vi "Make File Tree.vi"(8 "Error In":errorcluster, 10 "TreeControl in":refnum<vi>, 11 "WAD Main Cluster":T1) -> (0 "Error Out":errorcluster, 2 "TreeControl OUT":refnum<vi>, 3 "WAD Main Cluster OUT":T1)   [LabVIEW 2017]
uses:
  WAD_MainCluster.ctl
  TextureList.ctl
  PatchList.ctl
  Lumps.ctl
  <userlib>/_OpenG.lib/array/array.llb/Remove Duplicates from 1D Array (String)__ogtk.vi
  <userlib>/_OpenG.lib/array/array.llb/Filter 1D Array (String)__ogtk.vi
  <vilib>/regexp/Match Regular Expression.xnode
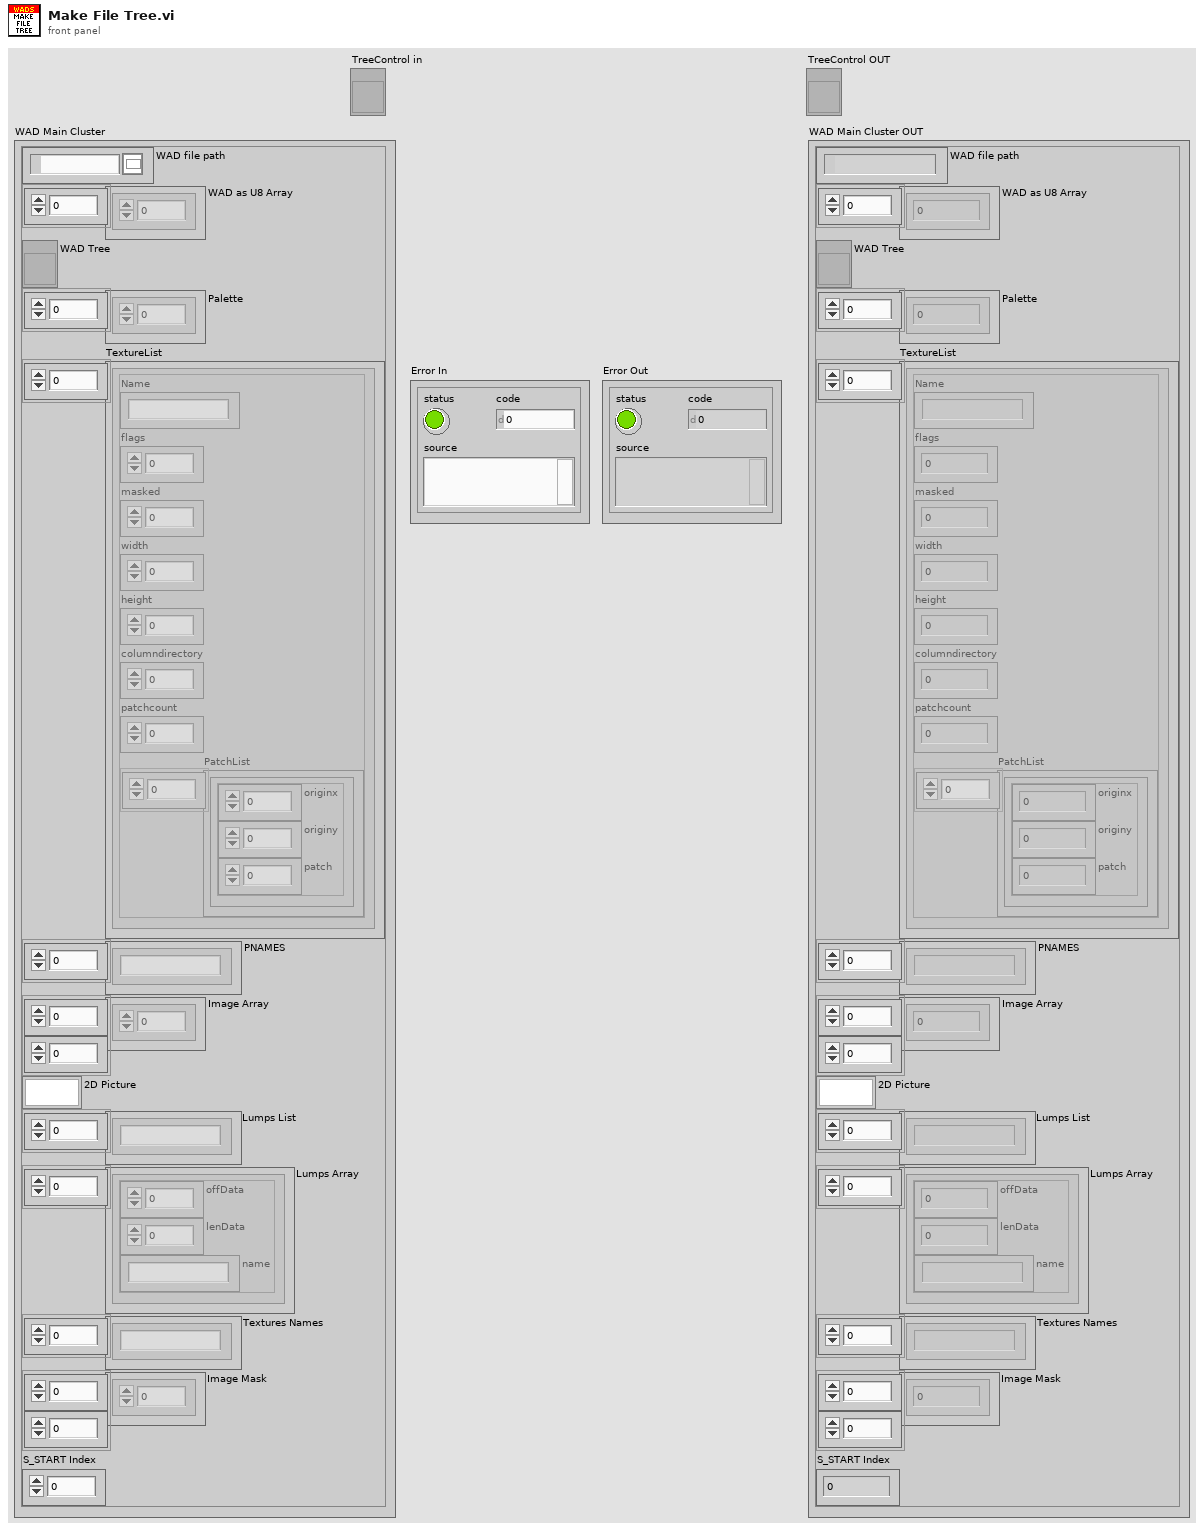
[diagram p1: front panel]
types:
  T1 = typedef "WAD_MainCluster.ctl" = cluster{"WAD file path":path, "WAD as U8 Array":u8[], "WAD Tree":refnum<vi>, "Palette":u32[], "TextureList":T2[], "PNAMES":string[], "Image Array":i16[][], "2D Picture":picture, "Lumps List":string[], "Lumps Array":T4[], "Textures Names":string[], "Image Mask":i16[][], "S_START Index":i32}
  T2 = typedef "TextureList.ctl" = cluster{"Name":string, "flags":u16, "masked":i16, "width":i16, "height":i16, "columndirectory":u32, "patchcount":i16, "PatchList":T3[]}
  T3 = typedef "PatchList.ctl" = cluster{"originx":i16, "originy":i16, "patch":i16}
  T4 = typedef "Lumps.ctl" = cluster{"offData":i32, "lenData":i32, "name":string}
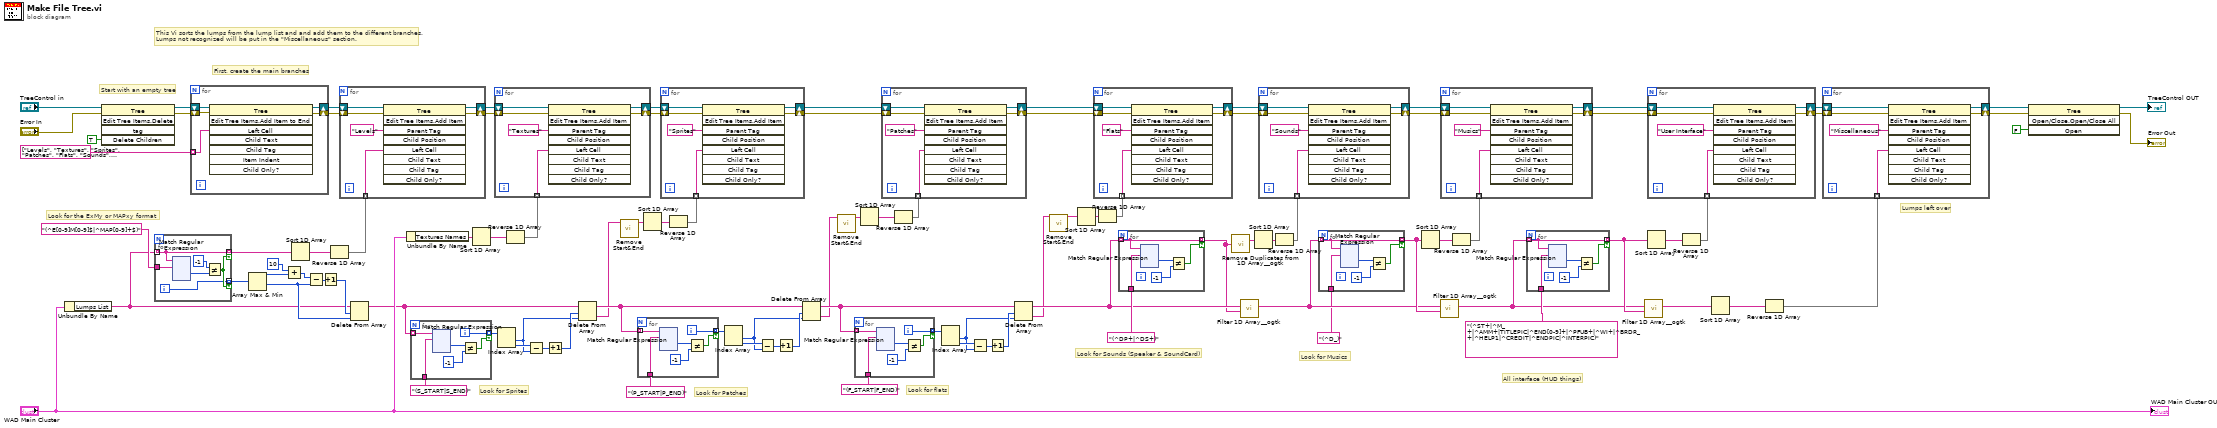
[diagram p0: block diagram]
diagram:
  # "This Vi sorts the lumps from the lump list and and add them to the different branches.\nLumps not recognized will be put in the \"Miscellaneous\" section."
  # "Start with an empty tree"
  # "First, create the main branches"
  # "Look for Musics"
  # "Lumps left over"
  # "All interface (HUD things)"
  # "Look for Sounds (Speaker & SoundCard)"
  # "Look for Sprites"
  # "Look for Patches"
  # "Look for flats"
  # "Look for the ExMy or MAPxy format"
  n1 = Unbundle By Name("WAD Main Cluster") -> ("Lumps List"=w5:string[])
  n2 = invoke on="Invoke Node" class="Tree" method="Edit Tree Items.Delete"(reference="TreeControl in", error in="Error In", "Delete Children"=TRUE ("Delete Children?")) -> (reference out=w90:refnum<vi>, error out=w92:errorcluster)  [unwired: 2 in, 3 out]
  n3 = for {
    tunnel: w5 -> [w101] mode=indexing
    tunnel: "(^E[0-9]M[0-9]$|^MAP[0-9]+$)" ("format string") -> [w102]
    tunnel: [w101] -> w83 mode=indexing if=w99
    tunnel: [w98] -> w65 mode=indexing if=w99
    i -> [w98]
    n4 = xnode "Match Regular Expression"("input string"=w101, "regular expression"=w102) -> ("offset past match"=w100:i32)  [unwired: 4 in, 4 out]
    n5 = Not Equal?(x=-1, y=w100) -> (x != y?=w99:bool)
  }
  n6 = for {
    tunnel: string[] ["Levels", "Textures", "Sprites", "Patches", "Flats", "Sounds", "Musics", "User Interface", "Miscellaneous"] -> [w220] mode=indexing
    shift-right: [w221] -> w93
    shift-left: w92 -> [w222]
    shift-right: [w218] -> w89
    shift-left: w90 -> [w219]
    n7 = invoke on="Invoke Node" class="Tree" method="Edit Tree Items.Add Item to End"(reference=w219, error in=w222, "Left Cell"=w220) -> (reference out=w218:refnum<vi>, error out=w221:errorcluster)  [unwired: 5 in, 6 out]
  }
  n8 = Array Max & Min(array=w65) -> (max value=w64:i32, min value=w61:i32)  [unwired: 2 out]
  n9 = Add(x=10, y=w64) -> (x+y=w62:i32)
  n10 = Sort 1D Array(array=w83) -> (sorted array=w14:string[])
  n11 = Subtract(x=w62, y=w61) -> (x-y=w60:i32)
  n12 = Increment(x=w60) -> (x+1=w59:i32)
  n13 = Reverse 1D Array(array=w14) -> (reversed array=w94:string[])
  n14 = for {
    tunnel: w94 -> [w223] mode=indexing
    shift-right: [w226] -> w32
    shift-left: w93 -> [w228]
    shift-right: [w224] -> w33
    shift-left: w89 -> [w225]
    n15 = invoke on="Invoke Node" class="Tree" method="Edit Tree Items.Add Item"(reference=w225, error in=w228, "Parent Tag"="Levels", "Left Cell"=w223) -> (reference out=w224:refnum<vi>, error out=w226:errorcluster)  [unwired: 5 in, 7 out]
  }
  n16 = Delete From Array(array=w5, length=w59, index=w61) -> (array with subset deleted=w58:string[])  [unwired: 1 out]
  n17 = Unbundle By Name("WAD Main Cluster") -> ("Textures Names"=w86:string[])
  n18 = for {
    tunnel: w58 -> [w231] mode=indexing
    tunnel: "(S_START|S_END)" ("format string") -> [w232]
    tunnel: [w229] -> w71 mode=indexing if=w230
    i -> [w229]
    n19 = xnode "Match Regular Expression"("input string"=w231, "regular expression"=w232) -> ("offset past match"=w234:i32)  [unwired: 4 in, 4 out]
    n20 = Not Equal?(x=w234, y=-1) -> (x != y?=w230:bool)
  }
  n21 = Sort 1D Array(array=w86) -> (sorted array=w13:string[])
  n22 = Index Array(array=w71) -> (element #1=w38:i32, element #2=w70:i32)  [unwired: 2 in]
  n23 = Reverse 1D Array(array=w13) -> (reversed array=w96:string[])
  n24 = for {
    shift-right: [w352] -> w30
    shift-left: w32 -> [w354]
    tunnel: w96 -> [w351] mode=indexing
    shift-right: [w349] -> w31
    shift-left: w33 -> [w350]
    n25 = invoke on="Invoke Node" class="Tree" method="Edit Tree Items.Add Item"(reference=w350, error in=w354, "Parent Tag"="Textures", "Left Cell"=w351) -> (reference out=w349:refnum<vi>, error out=w352:errorcluster)  [unwired: 5 in, 7 out]
  }
  n26 = Subtract(x=w70, y=w38) -> (x-y=w68:i32)
  n27 = Increment(x=w68) -> (x+1=w57:i32)
  n28 = Delete From Array(array=w58, length=w57, index=w38) -> (deleted portion=w27:string[], array with subset deleted=w56:string[])
  n29 = call "Remove Start&End.vi"("Lumps List"=w27) -> ("filtered array"=w26:string[])  [unwired: 10 in]
  n30 = for {
    tunnel: w56 -> [w357] mode=indexing
    tunnel: "(P_START|P_END)" ("format string") -> [w358]
    tunnel: [w355] -> w76 mode=indexing if=w356
    i -> [w355]
    n31 = xnode "Match Regular Expression"("input string"=w357, "regular expression"=w358) -> ("offset past match"=w360:i32)  [unwired: 4 in, 4 out]
    n32 = Not Equal?(x=w360, y=-1) -> (x != y?=w356:bool)
  }
  n33 = Sort 1D Array(array=w26) -> (sorted array=w12:string[])
  n34 = Reverse 1D Array(array=w12) -> (reversed array=w67:string[])
  n35 = for {
    shift-right: [w478] -> w24
    shift-left: w30 -> [w480]
    tunnel: w67 -> [w477] mode=indexing
    shift-right: [w475] -> w25
    shift-left: w31 -> [w476]
    n36 = invoke on="Invoke Node" class="Tree" method="Edit Tree Items.Add Item"(reference=w476, error in=w480, "Parent Tag"="Sprites", "Left Cell"=w477) -> (reference out=w475:refnum<vi>, error out=w478:errorcluster)  [unwired: 5 in, 7 out]
  }
  n37 = Index Array(array=w76) -> (element #1=w37:i32, element #2=w77:i32)  [unwired: 2 in]
  n38 = Subtract(x=w77, y=w37) -> (x-y=w74:i32)
  n39 = Increment(x=w74) -> (x+1=w46:i32)
  n40 = Delete From Array(array=w56, length=w46, index=w37) -> (deleted portion=w35:string[], array with subset deleted=w49:string[])
  n41 = call "Remove Start&End.vi"("Lumps List"=w35) -> ("filtered array"=w34:string[])  [unwired: 10 in]
  n42 = for {
    tunnel: w49 -> [w483] mode=indexing
    tunnel: "(F_START|F_END)" ("format string") -> [w484]
    tunnel: [w481] -> w81 mode=indexing if=w482
    i -> [w481]
    n43 = xnode "Match Regular Expression"("input string"=w483, "regular expression"=w484) -> ("offset past match"=w486:i32)  [unwired: 4 in, 4 out]
    n44 = Not Equal?(x=w486, y=-1) -> (x != y?=w482:bool)
  }
  n45 = Sort 1D Array(array=w34) -> (sorted array=w11:string[])
  n46 = Reverse 1D Array(array=w11) -> (reversed array=w73:string[])
  n47 = for {
    shift-right: [w604] -> w54
    shift-left: w24 -> [w606]
    tunnel: w73 -> [w603] mode=indexing
    shift-right: [w601] -> w55
    shift-left: w25 -> [w602]
    n48 = invoke on="Invoke Node" class="Tree" method="Edit Tree Items.Add Item"(reference=w602, error in=w606, "Parent Tag"="Patches", "Left Cell"=w603) -> (reference out=w601:refnum<vi>, error out=w604:errorcluster)  [unwired: 5 in, 7 out]
  }
  n49 = Index Array(array=w81) -> (element #1=w36:i32, element #2=w80:i32)  [unwired: 2 in]
  n50 = Subtract(x=w80, y=w36) -> (x-y=w79:i32)
  n51 = Increment(x=w79) -> (x+1=w47:i32)
  n52 = Delete From Array(array=w49, length=w47, index=w36) -> (deleted portion=w29:string[], array with subset deleted=w40:string[])
  n53 = call "Remove Start&End.vi"("Lumps List"=w29) -> ("filtered array"=w28:string[])  [unwired: 10 in]
  n54 = Sort 1D Array(array=w28) -> (sorted array=w10:string[])
  n55 = Reverse 1D Array(array=w10) -> (reversed array=w78:string[])
  n56 = for {
    shift-right: [w610] -> w52
    shift-left: w54 -> [w612]
    tunnel: w78 -> [w609] mode=indexing
    shift-right: [w607] -> w53
    shift-left: w55 -> [w608]
    n57 = invoke on="Invoke Node" class="Tree" method="Edit Tree Items.Add Item"(reference=w608, error in=w612, "Parent Tag"="Flats", "Left Cell"=w609) -> (reference out=w607:refnum<vi>, error out=w610:errorcluster)  [unwired: 5 in, 7 out]
  }
  n58 = for {
    tunnel: w40 -> [w614] mode=indexing
    tunnel: "(^DP+|^DS+)" ("format string") -> [w615]
    tunnel: [w614] -> w3 mode=indexing if=w613
    n59 = xnode "Match Regular Expression"("input string"=w614, "regular expression"=w615) -> ("offset past match"=w617:i32)  [unwired: 4 in, 4 out]
    n60 = Not Equal?(x=w617, y=-1) -> (x != y?=w613:bool)
  }
  n61 = call-poly <userlib>:"Remove Duplicates from 1D Array__ogtk.vi"("Input Array"=w3) -> ("Output Array"=w2:string[])  [unwired: 1 out]
  n62 = call-poly <userlib>:"Filter 1D Array__ogtk.vi"("items to filter"=w3, "array"=w40) -> ("filtered array"=w22:string[])  [unwired: 4 in, 1 out]
  n63 = Sort 1D Array(array=w2) -> (sorted array=w9:string[])
  n64 = Reverse 1D Array(array=w9) -> (reversed array=w4:string[])
  n65 = for {
    shift-right: [w735] -> w19
    shift-left: w52 -> [w737]
    tunnel: w4 -> [w734] mode=indexing
    shift-right: [w732] -> w20
    shift-left: w53 -> [w733]
    n66 = invoke on="Invoke Node" class="Tree" method="Edit Tree Items.Add Item"(reference=w733, error in=w737, "Parent Tag"="Sounds", "Left Cell"=w734) -> (reference out=w732:refnum<vi>, error out=w735:errorcluster)  [unwired: 5 in, 7 out]
  }
  n67 = for {
    tunnel: w22 -> [w739] mode=indexing
    tunnel: "(^D_)" ("format string") -> [w740]
    tunnel: [w739] -> w23 mode=indexing if=w738
    n68 = xnode "Match Regular Expression"("input string"=w739, "regular expression"=w740) -> ("offset past match"=w742:i32)  [unwired: 4 in, 4 out]
    n69 = Not Equal?(x=w742, y=-1) -> (x != y?=w738:bool)
  }
  n70 = Sort 1D Array(array=w23) -> (sorted array=w8:string[])
  n71 = call-poly <userlib>:"Filter 1D Array__ogtk.vi"("items to filter"=w23, "array"=w22) -> ("filtered array"=w15:string[])  [unwired: 4 in, 1 out]
  n72 = Reverse 1D Array(array=w8) -> (reversed array=w16:string[])
  n73 = for {
    shift-right: [w860] -> w17
    shift-left: w19 -> [w862]
    tunnel: w16 -> [w859] mode=indexing
    shift-right: [w857] -> w18
    shift-left: w20 -> [w858]
    n74 = invoke on="Invoke Node" class="Tree" method="Edit Tree Items.Add Item"(reference=w858, error in=w862, "Parent Tag"="Musics", "Left Cell"=w859) -> (reference out=w857:refnum<vi>, error out=w860:errorcluster)  [unwired: 5 in, 7 out]
  }
  n75 = for {
    tunnel: w15 -> [w864] mode=indexing
    tunnel: "(^ST+|^M_+|^AMM+|TITLEPIC|^END[0-9]+|^PFUB+|^WI+|^BRDR_+|^HELP1|^CREDIT|^ENDPIC|^INTERPIC)" ("format string") -> [w865]
    tunnel: [w864] -> w39 mode=indexing if=w863
    n76 = xnode "Match Regular Expression"("input string"=w864, "regular expression"=w865) -> ("offset past match"=w867:i32)  [unwired: 4 in, 4 out]
    n77 = Not Equal?(x=w867, y=-1) -> (x != y?=w863:bool)
  }
  n78 = call-poly <userlib>:"Filter 1D Array__ogtk.vi"("items to filter"=w39, "array"=w15) -> ("filtered array"=w42:string[])  [unwired: 4 in, 1 out]
  n79 = Sort 1D Array(array=w39) -> (sorted array=w6:string[])
  n80 = Reverse 1D Array(array=w6) -> (reversed array=w41:string[])
  n81 = for {
    shift-right: [w985] -> w45
    shift-left: w17 -> [w987]
    tunnel: w41 -> [w984] mode=indexing
    shift-right: [w982] -> w44
    shift-left: w18 -> [w983]
    n82 = invoke on="Invoke Node" class="Tree" method="Edit Tree Items.Add Item"(reference=w983, error in=w987, "Parent Tag"="User Interface", "Left Cell"=w984) -> (reference out=w982:refnum<vi>, error out=w985:errorcluster)  [unwired: 5 in, 7 out]
  }
  n83 = Sort 1D Array(array=w42) -> (sorted array=w7:string[])
  n84 = Reverse 1D Array(array=w7) -> (reversed array=w48:string[])
  n85 = for {
    shift-right: [w991] -> w50
    shift-left: w45 -> [w993]
    tunnel: w48 -> [w990] mode=indexing
    shift-right: [w988] -> w51
    shift-left: w44 -> [w989]
    n86 = invoke on="Invoke Node" class="Tree" method="Edit Tree Items.Add Item"(reference=w989, error in=w993, "Parent Tag"="Miscellaneous", "Left Cell"=w990) -> (reference out=w988:refnum<vi>, error out=w991:errorcluster)  [unwired: 5 in, 7 out]
  }
  n87 = invoke on="Invoke Node" class="Tree" method="Open/Close.Open/Close All"(reference=w51, error in=w50, "Open"=FALSE ("Open?")) -> (reference out=→"TreeControl OUT":refnum<vi>, error out=→"Error Out":errorcluster)  [unwired: 1 in, 2 out]
  "WAD Main Cluster OUT" <- "WAD Main Cluster"
